vi "Create Result.vi"(8 "error in (no error)":errorcluster, 11 "Experiment3D in":refnum<class "Experiment3D.lvclass">) -> (0 "error out":errorcluster, 2 "Text":string, 3 "Experiment3D out":refnum<class "Experiment3D.lvclass">)   [LabVIEW 2014, in "Experiment3D.lvclass"]
uses:
  Experiment3D.lvclass
  Data/Data3D/Data3D.lvclass
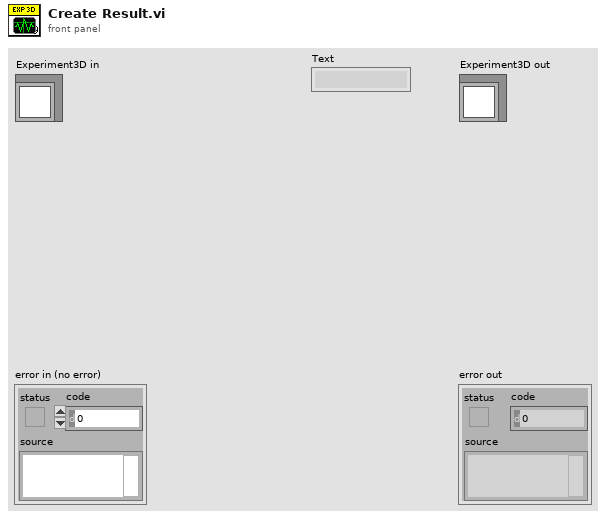
[diagram p1: front panel]
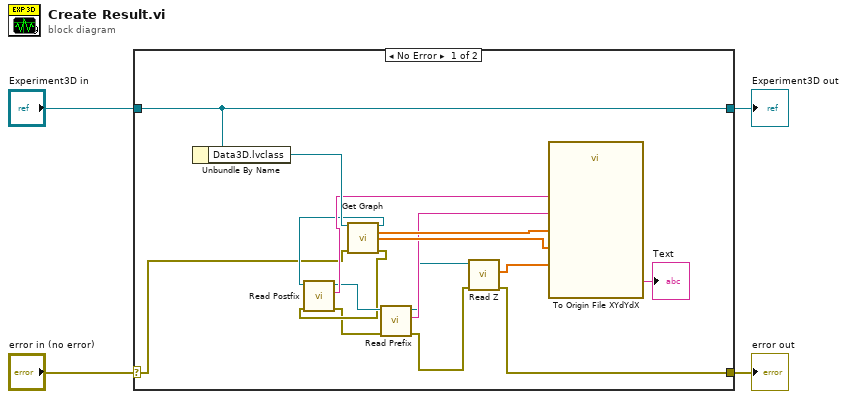
[diagram p0: block diagram]
diagram:
  n1 = case shown="No Error" "error in (no error)" {
    selector: "error in (no error)" -> [w9 w22]
    tunnel: [w5 w22] -> w3
    tunnel: [w20 w21] -> w1
    tunnel: "Experiment3D in" -> [w20 w21]
    frame No Error {
      n2 = Unbundle By Name(w20) -> ("Data3D.lvclass"=w19:refnum<class "Data3D.lvclass">)
      n3 = call "Get Graph.vi"("Data3D in"=w19, "error in (no error)"=w9) -> ("Data3D out"=w13:refnum<class "Data3D.lvclass">, "X"=w18:dbl[], "Y"=w17:dbl[], "error out"=w11:errorcluster)  [unwired: 9 in, 1 out]
      n4 = call "Read Postfix.vi"("error in (no error)"=w11, "Data3D in"=w13) -> ("error out"=w10:errorcluster, "Postfix"=w14:string, "Data3D out"=w12:refnum<class "Data3D.lvclass">)  [unwired: 7 in]
      n5 = call "Read Prefix.vi"("error in (no error)"=w10, "Data3D in"=w12) -> ("error out"=w6:errorcluster, "Prefix"=w15:string, "Data3D out"=w8:refnum<class "Data3D.lvclass">)  [unwired: 7 in]
      n6 = call "Read Z.vi"("error in (no error)"=w6, "Data3D in"=w8) -> ("error out"=w5:errorcluster, "Z"=w7:dbl[])  [unwired: 7 in, 1 out]
      n7 = call "To Origin File XYdYdX.vi"("Y"=w17, "dYdX"=w7, "X"=w18, "Postfix"=w14, "Prefix"=w15) -> ("Text"=→"Text":string)  [unwired: 6 in]
    }
    frame Error {
    }
  }
  "error out" <- w3
  "Experiment3D out" <- w1
